vi "mro apply Stock Command(incomplete).vi"(8 "error in (no error)":errorcluster, 9 "status":i32, 10 "trig":i8, 11 "index":i32) -> (0 "error out":errorcluster, 1 "status out":i32, 3 "function return":i8)   [LabVIEW 2016, in "mirao52e_32bit.lvlib"]
doc: "MIRAOEXPORT MroBoolean MIRAOCALL mro_applyStockCommand(\n int index,\n MroBoolean trig,\n int* status\n );"
uses:
  mirao52e_32bit.lvlib
  mirao52e.dll
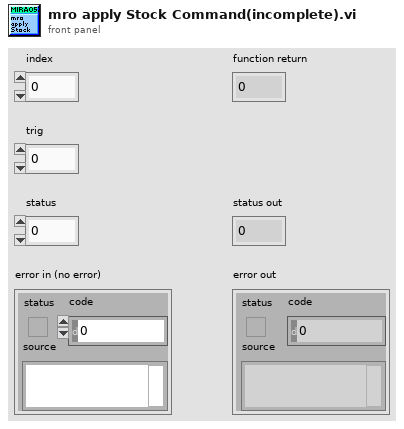
[diagram p1: front panel]
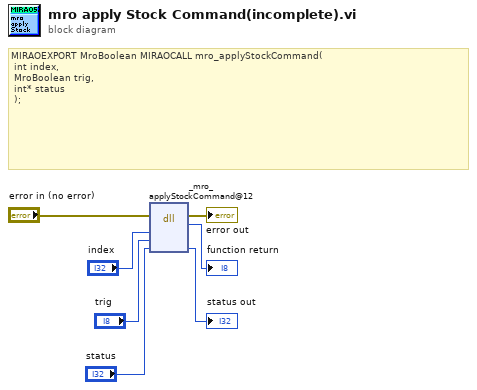
[diagram p0: block diagram]
diagram:
  # "MIRAOEXPORT MroBoolean MIRAOCALL mro_applyStockCommand(\n\tint index,\n\tMroBoolean trig,\n\tint* status\n\t);"
  n1 = dll-call lib="C:/Users/nvladim/Documents/Nikita-MDC/code/LabView/miraoDriver_32bit/mirao52e.*" fn="_mro_applyStockCommand@12"(error in="error in (no error)", "index"="index", "trig"="trig", "status"="status") -> (error out=→"error out":errorcluster, →"function return":i8, "status"=→"status out":i32)  [unwired: 4 in, 1 out]
